vi "TestOEPTiming.vi"() -> ()   [LabVIEW 2017]
uses:
  <vilib>/Platform/TimedLoop/XDataNode/timing_clust.ctl
  <vilib>/Platform/TimedLoop/XDataNode/nitl_modes.ctl
  <vilib>/Platform/TimedLoop/XDataNode/wakeup.ctl
  <vilib>/DAQmx/write.llb/DAQmx Write (Analog DBL 1Chan 1Samp).vi
  <vilib>/DAQmx/create/channels.llb/DAQmx Create Channel (AO-Voltage-Basic).vi
  <vilib>/DAQmx/configure/timing.llb/DAQmx Timing (Sample Clock).vi
  <vilib>/DAQmx/miscellaneous.llb/DAQmx Fill In Error Info.vi
  <vilib>/addons/zeromq/zmq_recv_multi.vi
  <vilib>/addons/zeromq/zmq_socket.lvclass
  <vilib>/platform/TimedLoop/XDataNode/XDataNode.xnode
  <vilib>/Platform/TimedLoop/XDataNode/XDNodeRunTimeDep.lvlib
  <vilib>/Analysis/NI_AALBase.lvlib
  kernel32.dll
  <vilib>/Analysis/NI_AALPro.lvlib
panel:
  in  "max":dbl format="%#_13g"
  in  "min":dbl=40.0 format="%#_13g"
  out "pulse-to-OEP time series":dbl(graph)
  out "ts 3":i64
  out "ts 2":i64
  out "ts 1":i64
  in  "Processor":i32=2
  out "ZMQ error":errorcluster
  in  "Start high":bool
  out "OEP-to-LV delay (ms)":T1(graph)
  in  "plot 2 bins":i32=10
  in  "Loop frequency (Hz)":dbl=5.0
  in  "TTL channel":u16=1 min=1 max=8
  in  "TTL port":u16=5557
  in  "?":bool
  in  "amplitude (V)":dbl=0.05 format="%#_13g"
  in  "AO physical channels":tag="pciDAQ/ao2"
  out "loop error":string=" INSTRUCTIONS:\r\rNormal Use:  When using subVIs that incorporate the error in/error out (or error I/O) structure, place this handler where you want to inform the user of an error, typically at the end of the I/O data path, as the last action of the program.  If the error in error? is ERROR, the handler creates a message describing the error and its source.  If the type of dialog = 1 (default), the message is displayed to the user, who can only acknowedge it.  If the type = 2, the user can acknowledge the message or abort execution; aborting a program with active I/O is not recommended.  If the type = 0, no message is displayed; this is used to process the error programmatically, and the error out cluster elements are wired to individual terminals for that reason.  \r\rOther Use:\n\r\nlocal testing.  To test the error code of a subVI or function that does not have the error I/O structure, you can wire its error code and a source string to the local error code and error source inputs.  If error in error? indicates no error and error code is not equal to 0, the local code and source are substituted for the error in values, and error? is set TRUE (ERROR)."
  in  "plot 1 bins":i32=10
  out "pulse-to-OEP delay":T1(graph)
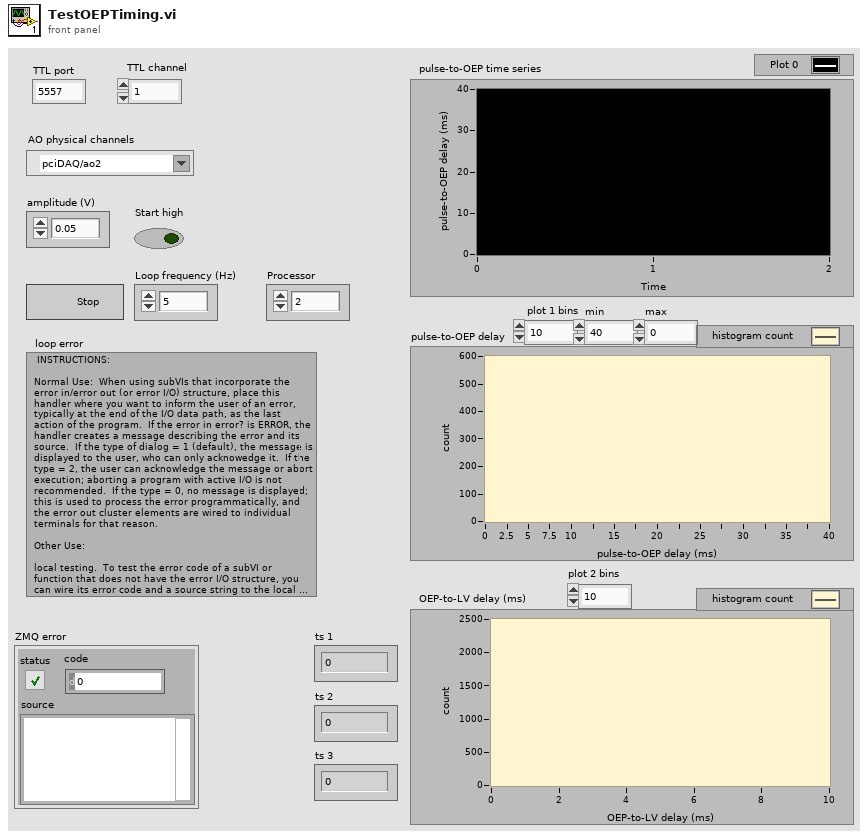
[diagram p1: front panel]
types:
  T1 = cluster{"X Values":dbl[], "Histogram: h(x)":i32[]}
  T2 = typedef "XDNodeRunTimeDep.lvlib/timing_clust.ctl" = cluster{"Expected End [f-1]":u64, "Actual End [f-1]":u64, "Finished Late? [f-1]":bool, "Expected End [i-1]":u64, "Actual End [i-1]":u64, "Finished Late? [i-1]":bool, "Expected Start [i]":u64, "Actual Start [i]":u64, "Expected Start [f]":u64, "Actual Start [f]":u64, "Source Name":string, "Structure Name":string, "Period":i64, "Deadline":i64, "Offset":i64, "Start":i64, "Priority":i32, "Timeout":i32, "Mode":T3, "Wakeup Reason":T4, "Error":errorcluster, "Source Type":string, "Secondary Source Type":string, "Global End Time":u64, "Global Start Time":u64, "Frame Duration":u64, "Iteration Duration":u64, "Assigned CPU":i32, "I/O Scan Engine Mode":u32}
  T3 = typedef "XDNodeRunTimeDep.lvlib/nitl_modes.ctl" = enum32{"No Change", "Process missed periods, maintain original phase", "Discard missed periods, maintain original phase", "Process missed periods, ignore original phase", "Discard missed periods, ignore original phase"}
  T4 = typedef "XDNodeRunTimeDep.lvlib/wakeup.ctl" = enum32{"Normal", "Aborted", "Asynchronous wakeup", "Timing source error", "Timed loop error", "Timeout"}
  T5 = enum16{"big-endian, network order", "native, host order", "little-endian"}
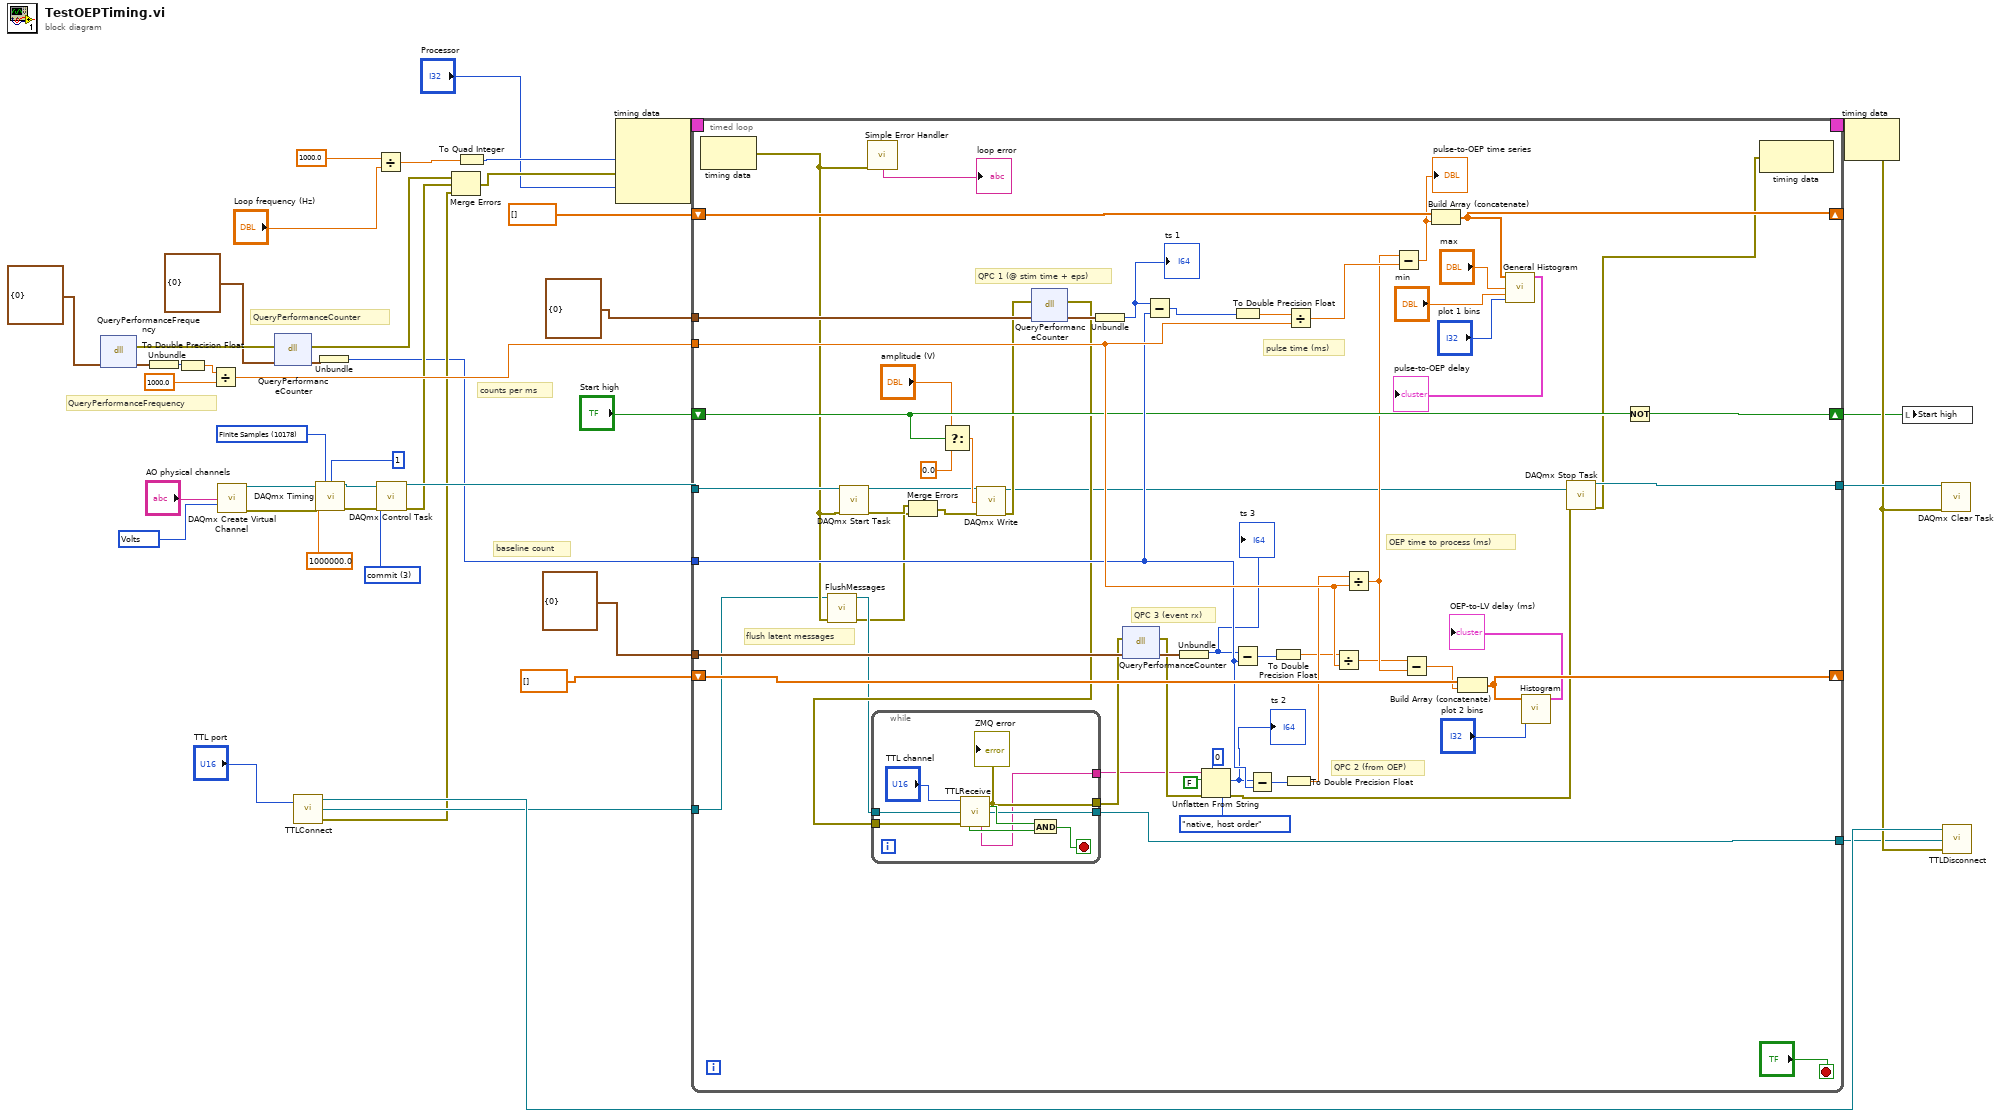
[diagram p0: block diagram]
diagram:
  w9 = 3 items=["verify"=2, "reserve"=4, "commit"=3, "unreserve"=5, "abort"=6] ("action")
  w28 = 10178 items=["Finite Samples"=10178, "Continuous Samples"=10123, "Hardware Timed Single Point"=12522] ("sample mode")
  w39 = 10348 items=["Volts"=10348, "From Custom Scale"=10065] ("units")
  # "QueryPerformanceCounter"
  # "baseline count"
  # "counts per ms"
  # "QueryPerformanceFrequency"
  n1 = dll-call lib="kernel32.dll" fn="QueryPerformanceFrequency"("lpFrequency"=cluster{i64} {0}) -> (error out=w8:errorcluster, "lpFrequency"=w41:cluster{i64})  [unwired: 4 in, 1 out]
  n2 = Unbundle(w41) -> (w23:i64)
  n3 = To Double Precision Float(number=w23) -> (double precision float=w21:dbl)
  n4 = Divide(x=w21, y=1000.0) -> (x/y=w20:dbl)
  n5 = call-poly <vilib>:"DAQmx Create Virtual Channel.vi"("physical channels"="AO physical channels", "units"=w39) -> ("task out"=w24:refnum<k21>, "error out"=w27:errorcluster)  [unwired: 12 in]
  n6 = dll-call lib="kernel32.dll" fn="QueryPerformanceCounter"(error in=w8, cluster{i64} {0}) -> (error out=w6:errorcluster, w4:cluster{i64})  [unwired: 3 in, 1 out]
  n7 = call "TTLConnect.vi"("port"="TTL port") -> ("context out"=w37:refnum<class "zmq_context.lvclass">, "socket out"=w36:refnum<class "zmq_socket.lvclass">, "error out"=w16:errorcluster)  [unwired: 1 in]
  n8 = call-poly <vilib>:"DAQmx Timing.vi"("task/channels in"=w24, "sample mode"=w28, "samples per channel"=1, "rate"=1000000.0, "error in"=w27) -> ("task out"=w19:refnum<k21>, "error out"=w25:errorcluster)  [unwired: 9 in]
  n9 = Unbundle(w4) -> (w5:i64)
  n10 = Divide(x=1000.0, y="Loop frequency (Hz)") -> (x/y=w35:dbl)
  n11 = call <vilib>:"DAQmx Control Task.vi"("task/channels in"=w19, "action"=w9, "error in"=w25) -> ("task out"=w26:refnum<k21>, "error out"=w17:errorcluster)  [unwired: 11 in]
  n12 = Merge Errors(w6, w17, w16) -> (w18:errorcluster)
  n13 = To Quad Integer(1:w35) -> (0:w34:i64)
  n14 = node-c288(w34, w18, "Processor") -> (w44:T2)  [unwired: 1 in]
  n15 = timed-loop {
    timing: w44 -> [_]
    timing-out: [_] -> w43
    shift-right: [w100] -> _
    shift-left: dbl[] [] -> [w102]
    tunnel: w26 -> [w93]
    tunnel: [w92] -> w31
    tunnel: w36 -> [w52]
    tunnel: w20 -> [w96]
    tunnel: cluster{i64} {0} -> [w98]
    tunnel: cluster{i64} {0} -> [w97]
    shift-right: [w94] -> _
    shift-left: dbl[] [] -> [w95]
    tunnel: w5 -> [w91]
    shift-right: [w90] -> w2
    shift-left: "Start high" -> [w89]
    tunnel: [w87] -> w1
    stop <- "?" stop-if-true
    # "flush latent messages"
    # "QPC 3 (event rx)"
    # "OEP time to process (ms)"
    # "QPC 2 (from OEP)"
    # "pulse time (ms)"
    # "QPC 1 (@ stim time + eps)"
    n16 = node-c288() -> (w53:errorcluster)  [unwired: 1 in]
    n17 = call "FlushMessages.vi"("error in (no error)"=w53, "zmq_socket in"=w52) -> ("error out"=w48:errorcluster, "zmq_socket out"=w51:refnum<class "zmq_socket.lvclass">)  [unwired: 8 in]
    n18 = call <vilib>:"DAQmx Start Task.vi"("task/channels in"=w93, "error in"=w53) -> ("task out"=w63:refnum<k21>, "error out"=w49:errorcluster)  [unwired: 12 in]
    n19 = call <vilib>:"Simple Error Handler.vi"("error in (no error)"=w53) -> ("message"=→"loop error":string)  [unwired: 4 in, 4 out]
    n20 = Merge Errors(w49, w48) -> (w50:errorcluster)
    n21 = Select(t="amplitude (V)", s=w89, f=0.0) -> (s? t:f=w76:dbl)
    n22 = call-poly <vilib>:"DAQmx Write.vi"("task/channels in"=w63, "data"=w76, "error in"=w50) -> ("task out"=w62:refnum<k21>, "error out"=w75:errorcluster)  [unwired: 10 in, 1 out]
    n23 = dll-call lib="kernel32.dll" fn="QueryPerformanceCounter"(error in=w75, w98) -> (error out=w64:errorcluster, w84:cluster{i64})  [unwired: 3 in, 1 out]
    n24 = while {
      tunnel: w51 -> [w111]
      tunnel: [w106] -> w87
      tunnel: [w105] -> w73
      tunnel: [w104] -> w57
      tunnel: w64 -> [w103]
      stop <- w109 stop-if-true
      n25 = call "TTLReceive.vi"("channel"="TTL channel", "socket in"=w111, "error in"=w103) -> ("new TTL"=w107:bool, "socket out"=w106:refnum<class "zmq_socket.lvclass">, "event on"=w108:bool, "metadata"=w104:string, "error out"=w105:errorcluster)  [unwired: 7 in, 1 out]
      "ZMQ error" <- w105
      n26 = And(x=w107, y=w108) -> (x .and. y?=w109:bool)
    }
    n27 = Unbundle(w84) -> (w56:i64)
    "ts 1" <- w56
    n28 = dll-call lib="kernel32.dll" fn="QueryPerformanceCounter"(error in=w73, w97) -> (error out=w65:errorcluster, w72:cluster{i64})  [unwired: 3 in, 1 out]
    n29 = Subtract(x=w56, y=w91) -> (x-y=w61:i64)
    n30 = Unbundle(w72) -> (w55:i64)
    "ts 3" <- w55
    n31 = Unflatten From String(type=i64 0, binary string=w57, data includes array or string size? (T)=FALSE, byte order (0:big-endian, network order)=T5."native, host order", error in (no error)=w65) -> (value=w58:i64, error out=w54:errorcluster)  [unwired: 1 out]
    "ts 2" <- w58
    n32 = To Double Precision Float(number=w61) -> (double precision float=w83:dbl)
    n33 = Subtract(x=w55, y=w91) -> (x-y=w60:i64)
    n34 = Subtract(x=w58, y=w91) -> (x-y=w59:i64)
    n35 = To Double Precision Float(number=w60) -> (double precision float=w70:dbl)
    n36 = To Double Precision Float(number=w59) -> (double precision float=w74:dbl)
    n37 = Divide(x=w83, y=w96) -> (x/y=w77:dbl)
    n38 = Divide(x=w70, y=w96) -> (x/y=w69:dbl)
    n39 = Divide(x=w74, y=w96) -> (x/y=w71:dbl)
    n40 = Subtract(x=w71, y=w77) -> (x-y=w47:dbl)
    "pulse-to-OEP time series" <- w47
    n41 = Subtract(x=w69, y=w71) -> (x-y=w68:dbl)
    n42 = Build Array (concatenate)(w102, w47) -> (w100:dbl[])
    n43 = Build Array (concatenate)(w95, w68) -> (w94:dbl[])
    n44 = call <vilib>:"General Histogram.vi"("X"=w100, "max"="max", "min"="min", "# bins"="plot 1 bins") -> ("Histogram Graph"=→"pulse-to-OEP delay":T1)  [unwired: 7 in, 4 out]
    n45 = call <vilib>:"Histogram.vi"("intervals"="plot 2 bins", "X"=w94) -> ("Histogram Graph"=→"OEP-to-LV delay (ms)":T1)  [unwired: 6 in, 3 out]
    n46 = call <vilib>:"DAQmx Stop Task.vi"("task/channels in"=w62, "error in"=w54) -> ("task out"=w92:refnum<k21>, "error out"=w88:errorcluster)  [unwired: 12 in]
    n47 = Not(x=w89) -> (.not. x?=w90:bool)
    n48 = node-c288(w88) -> ()  [unwired: 1 out]
  }
  n49 = node-c288(w43) -> (w14:errorcluster)
  n50 = local write "Start high"(w2) -> ()
  n51 = call <vilib>:"DAQmx Clear Task.vi"("task in"=w31, "error in"=w14) -> ()  [unwired: 13 in, 1 out]
  n52 = call "TTLDisconnect.vi"("error in"=w14, "socket in"=w1, "context in"=w37) -> ()  [unwired: 1 in, 1 out]
